vi "Map 8CH Loopback to VS Channels.vi"(11 "Base Path to Ports":string) -> (0 "Channel Count":dbl[](array[numeric]), 1 "Rx Channel Array":string[](array[string]), 2 "Disable Channel Array":string[](array[string]), 3 "Tx Channel Array":string[](array[string]))   [LabVIEW 2020, in "Single Core Simple Loopback.lvclass"]
uses:
  Single Core Simple Loopback.lvclass
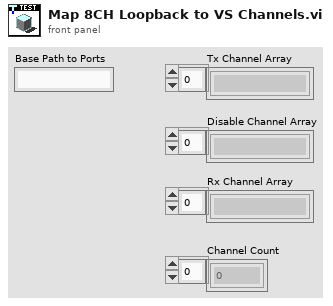
[diagram p1: front panel]
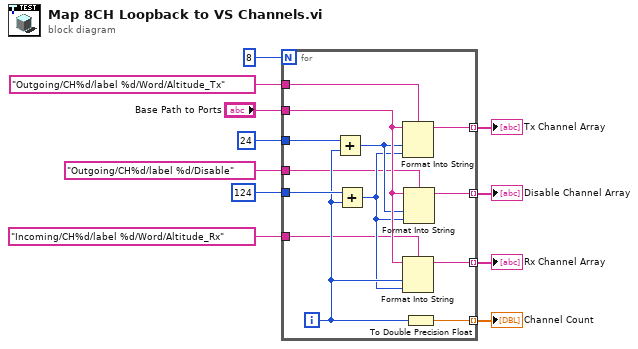
[diagram p0: block diagram]
diagram:
  n1 = for {
    N: 8 -> [_]
    tunnel: 24 ("x") -> [w24]
    tunnel: [w23] -> w8 mode=indexing
    tunnel: [w22] -> w9 mode=indexing
    tunnel: [w21] -> w7 mode=indexing
    tunnel: 124 ("x") -> [w20]
    tunnel: "Base Path to Ports" -> [w18]
    tunnel: [w15] -> w4 mode=indexing
    tunnel: "Outgoing/CH%d/label %d/Word/Altitude_Tx" ("format string") -> [w14]
    tunnel: "Outgoing/CH%d/label %d/Disable" ("format string") -> [w13]
    tunnel: "Incoming/CH%d/label %d/Word/Altitude_Rx" ("format string") -> [w12]
    i -> [w19]
    n2 = Add(x=w24, y=w19) -> (x+y=w17:i32)
    n3 = Add(x=w20, y=w19) -> (x+y=w16:i32)
    n4 = Format Into String(format string=w14, initial string=w18, w17, w16) -> (resulting string=w23:string)  [unwired: 1 in, 1 out]
    n5 = Format Into String(format string=w12, initial string=w18, w19, w16) -> (resulting string=w22:string)  [unwired: 1 in, 1 out]
    n6 = Format Into String(format string=w13, initial string=w18, w17, w16) -> (resulting string=w15:string)  [unwired: 1 in, 1 out]
    n7 = To Double Precision Float(number=w19) -> (double precision float=w21:dbl)
  }
  "Rx Channel Array" <- w9
  "Tx Channel Array" <- w8
  "Channel Count" <- w7
  "Disable Channel Array" <- w4
